vi "Set_Output_State.vi"(3 "rest off?":bool, 4 "error in":errorcluster, 5 "channel":u8=2 min=2 max=13 step=1, 6 "state":bool=TRUE, 7 "VISA arduino in":refnum<visa-resource-name>) -> (0 "error out":errorcluster, 1 "VISA arduino out":refnum<visa-resource-name>)   [LabVIEW 2021]
uses:
  <vilib>/Utility/error.llb/Error Cluster From Error Code.vi
  <vilib>/ErrorRing/Error Ring.xnode
panel:
  out "delay":u32
  # "Private"
  # "Public"
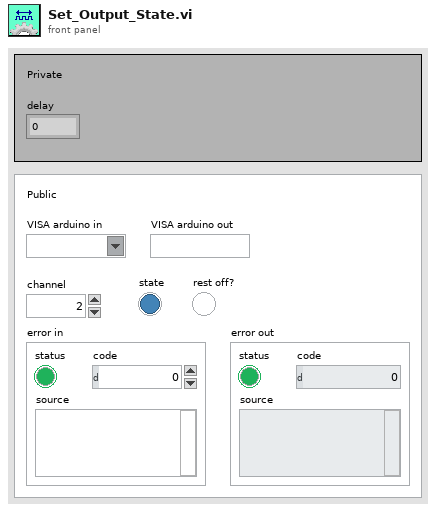
[diagram p1: front panel]
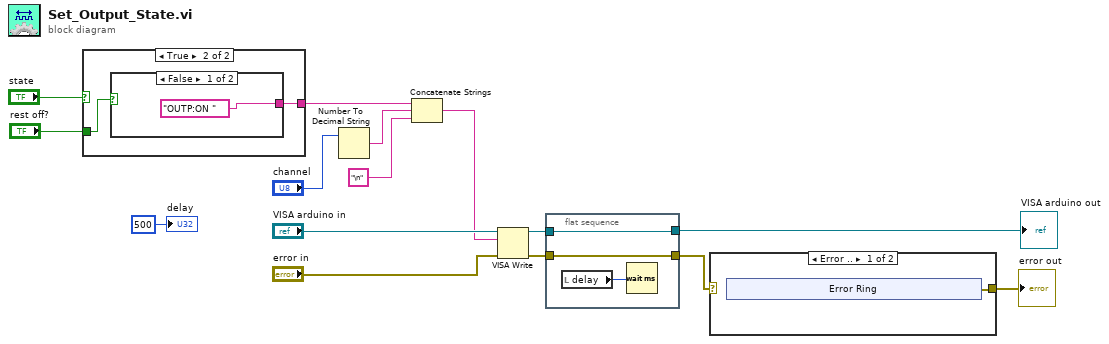
[diagram p0: block diagram]
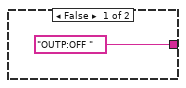
[diagram p3: hidden frame]
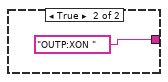
[diagram p4: hidden frame]
diagram:
  n1 = case shown="True" "state" {
    tunnel: "rest off?" -> [_ w18]
    tunnel: ["OUTP:OFF " w17] -> w11
    frame False {
    }
    frame True {
      n2 = case shown="False" w18 {
        tunnel: ["OUTP:ON " "OUTP:XON "] -> w17
        frame False {
        }
        frame True {
        }
      }
    }
  }
  n3 = Number To Decimal String(number="channel") -> (decimal integer string=w10:string)  [unwired: 1 in]
  n4 = Concatenate Strings(w11, w10, "\n" ("string")) -> (w6:string)
  n5 = VISA Write(VISA resource name="VISA arduino in", write buffer=w6, error in (no error)="error in") -> (VISA resource name out=w5:refnum<visa-resource-name>, error out=w4:errorcluster)  [unwired: 1 out]
  n6 = flat-sequence {
    tunnel: w5 -> [w22]
    tunnel: w4 -> [w21]
    tunnel: [w22] -> w2
    tunnel: [w21] -> w3
    frame #0 {
      n7 = local read "delay"() -> (w23:u32)
      n8 = Wait (ms)(milliseconds to wait=w23) -> ()  [unwired: 1 out]
    }
  }
  n9 = case shown="Error .." w3 {
    selector: w3 -> [_ w30]
    tunnel: [w24 w30] -> w1
    frame Error {
      n10 = xnode "Error Ring"() -> ("error out"=w24:errorcluster)
    }
    frame No Error {
    }
  }
  "error out" <- w1
  "delay" <- u32 500
  "VISA arduino out" <- w2
